vi "fft_demodulator.vi"(0 "Reset":bool, 5 "Config":T2={"IO params"={"Conversion"={"Rate"=4.0, "In channels"=2, "Out channels"=4}, "Carriers"={"Phase shift"=180.0, "Levels"=[[0.8, 0.8, 0.8], [0.03, 0.03, 0.03]], "Delay samples"=73.15}}, "High rate STFT"={"Win param"=101.5, "Window type"=61, "Win order"=2, "DFT size"=64, "Channels"=[7], "Oversample"=64}, "Low rate STFT"={"Win param"=120.0, "Window type"=61, "Win order"=8, "DFT size"=64, "Channels"=[7], "Oversample"=64}, "Filtering"={"Hum"={"Frequency"=0.0, "Tc"=0.0, "Limit"=101.5, "FFT filter"=FALSE, "Detrend mode"=enum."Robust linear", "Enable"=FALSE}, "Kalman"={"Process noise"=101.5, "Measure noise"=101.5, "Unlock m noise"=101.5, "Mode"=enum."FFT"}, "Distortion"={"LF cut"=101.5, "Tc"=3.0, "Limit"=101.5, "FFT filter"=FALSE, "Detrend mode"=enum."Robust linear", "Enable"=FALSE}, "Lowpass"={"Frequency"=0.0, "Order"=0, "Enable"=FALSE}, "Impulse"={"Win order"=102, "Locked limit"=101.5, "Locked count"=102, "Threshold Tc"=101.5, "Thresh sigmas"=101.5, "Thresh min"=101.5, "After"=0, "Detrend"=FALSE, "Enable"=FALSE}}} {"Filtering"."Impulse"."Thresh min" format="%#_3p"; "Filtering"."Impulse"."Threshold Tc" format="%#_3p"; "Filtering"."Impulse"."Locked limit" format="%#_3p"; "Filtering"."Impulse"."Thresh sigmas" format="%#_3p"; "Filtering"."Lowpass"."Frequency" format="%#_4p"; "Filtering"."Distortion"."Limit" format="%#_3p"; "Filtering"."Distortion"."LF cut" format="%#_3p"; "Filtering"."Kalman"."Unlock m noise" format="%#_3p"; "Filtering"."Kalman"."Measure noise" format="%#_3p"; "Filtering"."Kalman"."Process noise" format="%#_3p"; "Filtering"."Hum"."Limit" format="%#_3p"; "Filtering"."Hum"."Frequency" format="%#_4p"; "Low rate STFT"."Oversample" min=1 step=1; "Low rate STFT"."Channels" min=0 step=1; "Low rate STFT"."DFT size" min=1 step=1; "Low rate STFT"."Window type" items=["Rectangle"=0, "Hanning"=1, "Hamming"=2, "Blackman-Harris"=3, "Exact Blackman"=4, "Blackman"=5, "Flat Top"=6, "4 Term B-Harris "=7, "7 Term B-Harris"=8, "Low Sidelobe"=9, "Blackman Nuttall"=11, "Triangle"=30, "Bartlett-Hanning"=31, "Bohman"=32, "Parzen"=33, "Welch"=34, "Kaiser"=60, "Dolph-Chebyshev"=61, "Gaussian"=62]; "High rate STFT"."Oversample" min=1 step=1; "High rate STFT"."Channels" min=0 step=1; "High rate STFT"."DFT size" min=1 step=1; "High rate STFT"."Window type" items=["Rectangle"=0, "Hanning"=1, "Hamming"=2, "Blackman-Harris"=3, "Exact Blackman"=4, "Blackman"=5, "Flat Top"=6, "4 Term B-Harris "=7, "7 Term B-Harris"=8, "Low Sidelobe"=9, "Blackman Nuttall"=11, "Triangle"=30, "Bartlett-Hanning"=31, "Bohman"=32, "Parzen"=33, "Welch"=34, "Kaiser"=60, "Dolph-Chebyshev"=61, "Gaussian"=62]; "IO params"."Carriers"."Levels" min=0.0 step=0.1; "IO params"."Conversion"."Rate" format="%#_8g"}, 7 "Modulation info":T8={"Fs full"=0.0, "Fs high"=0.0, "Fs low"=0.0, "Read size"=0, "FFT size low"=5000, "df low"=5000.0, "High carriers"=[], "Low carriers"=[], "Hi channels at low"=[7]} {"Hi channels at low" min=0 step=1; "Low carriers" format="%#_6p"; "High carriers" format="%#_6p"}, 9 "Low carrier amplitudes":cdb[](array[numeric]) format="%#_3p", 12 "Raw data":dbl[](array[numeric])) -> (10 "High carrier amplitudes":cdb[][](array[numeric]) format="%_3p", 14 "Filtered signal":dbl[](array[numeric]), 15 "Trace channel out":T1)   [LabVIEW 2014]
uses:
  modulation_info.ctl
  ilemt_config.ctl
  IO_params.ctl
  stft_params.ctl
  <vilib>/Analysis/4window.llb/windowTd.ctl
  filter_params.ctl
  detrend_mode.ctl
  trace_channel.ctl
  <vilib>/Analysis/NI_AALPro.lvlib
panel:
  out "DIstortion filter attenuation":dbl
  out "Distortion filter RMS":dbl[](array[numeric])
  out "KF result":cdb[](array[numeric]) format="%_3p"
  out "Distortion filter":dbl[][](graph)
  # "This VI deals with high-rate demodulation and filtering for a single sensor axis."
  # "Rows are time (high carrier samples), columns are high rate source XYZ axis amplitudes."
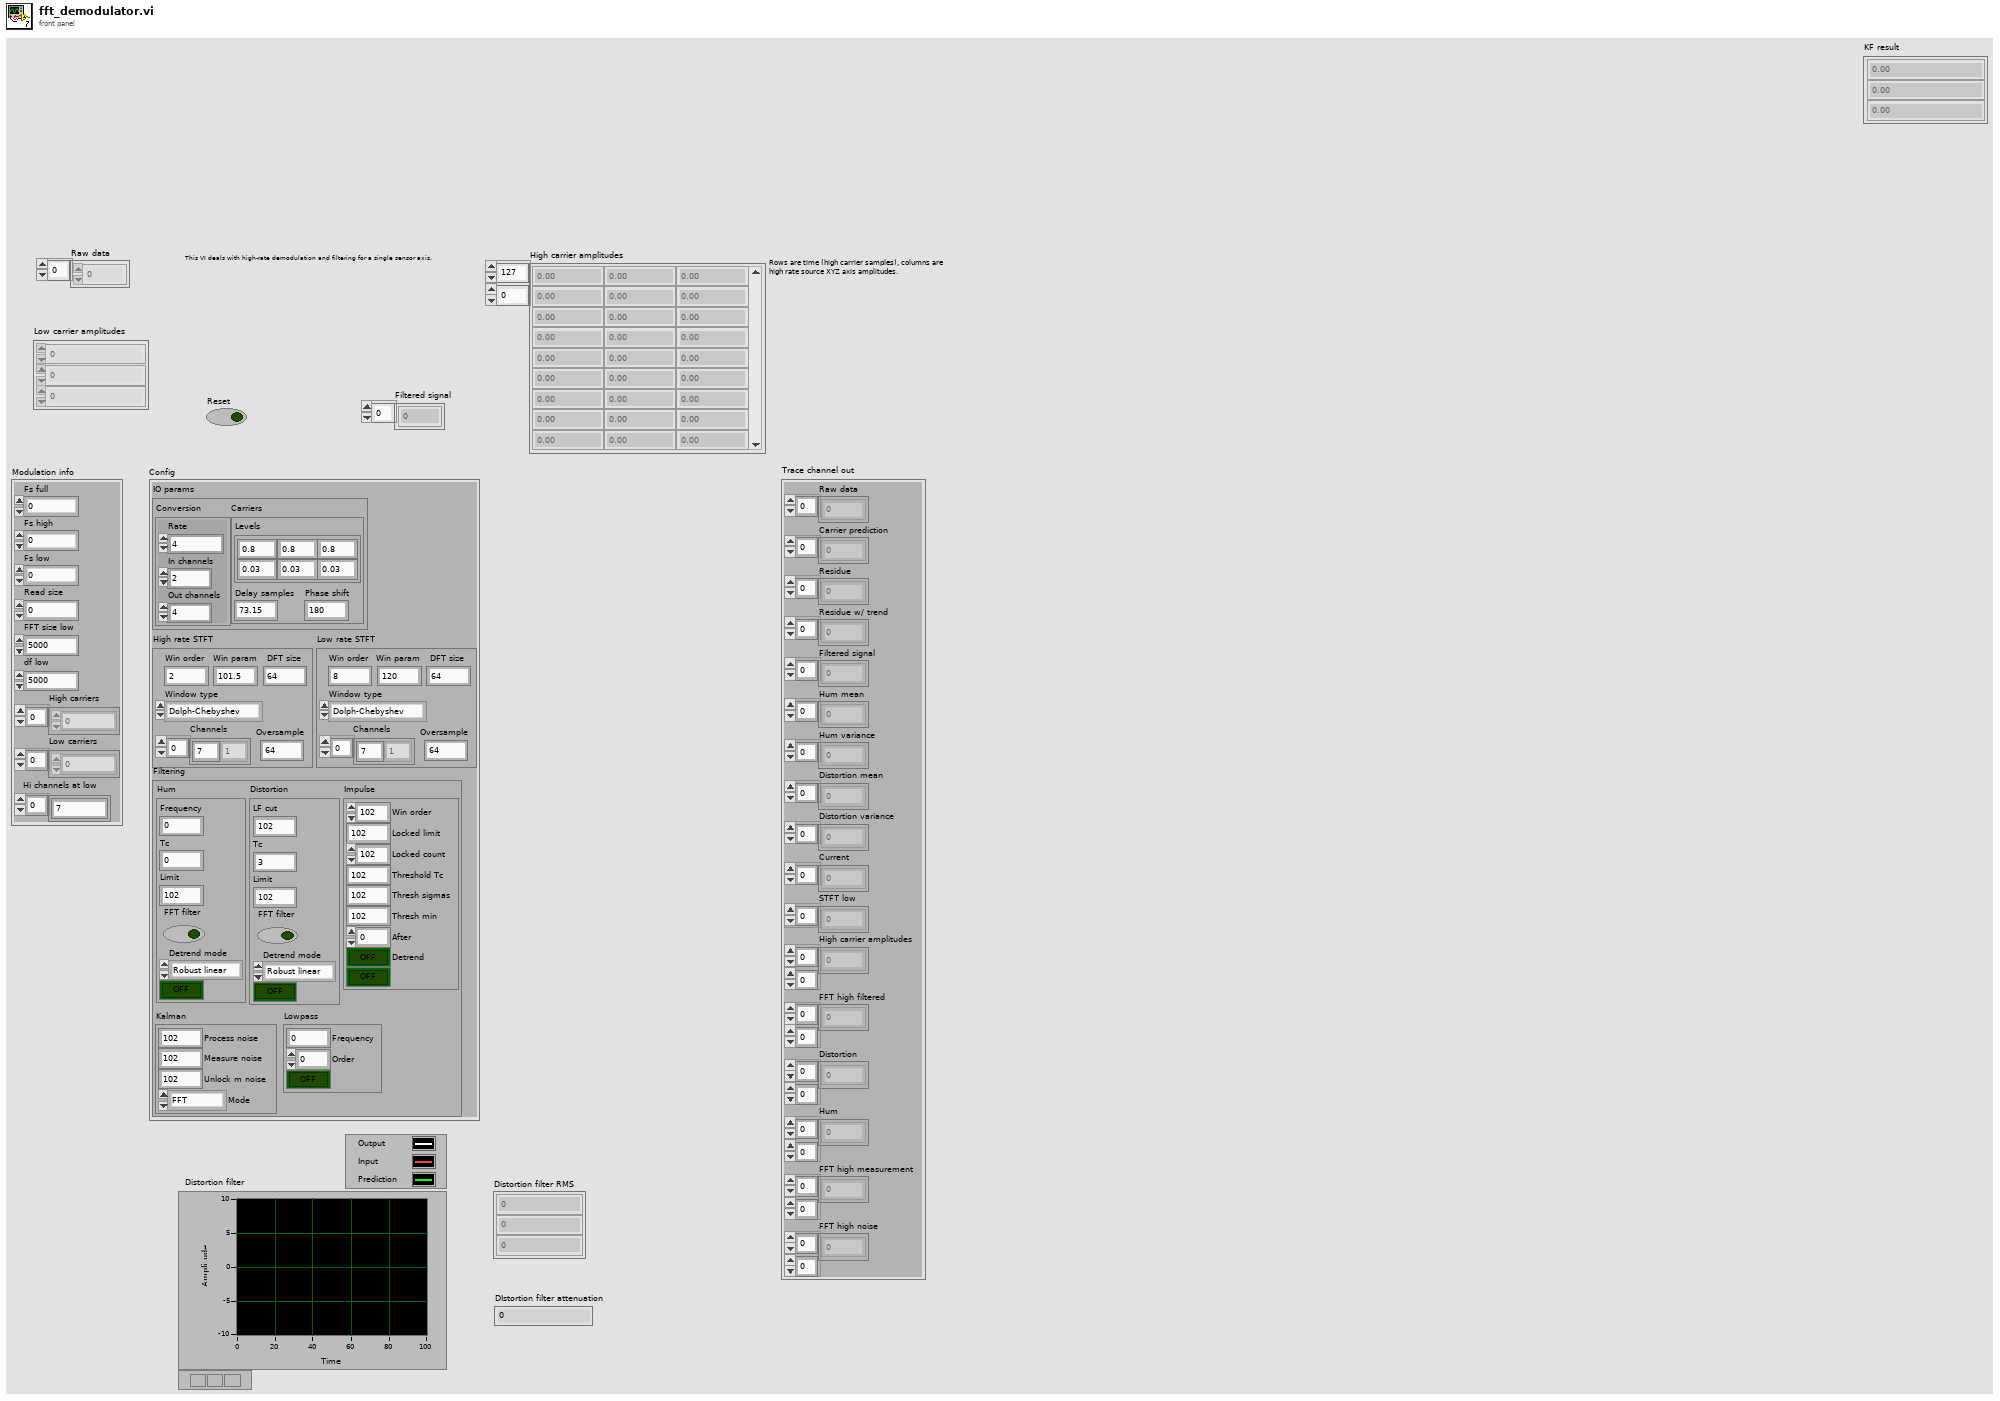
[diagram p1: front panel]
types:
  T1 = typedef "trace_channel.ctl" = cluster{"Raw data":dbl[], "Carrier prediction":dbl[], "Residue":dbl[], "Residue w/ trend":dbl[], "Filtered signal":dbl[], "Hum mean":dbl[], "Hum variance":dbl[], "Distortion mean":dbl[], "Distortion variance":dbl[], "Current":dbl[], "STFT low":cdb[], "High carrier amplitudes":cdb[][], "FFT high filtered":cdb[][], "Distortion":cdb[][], "Hum":cdb[][], "FFT high measurement":cdb[][], "FFT high noise":dbl[][]}
  T2 = typedef "ilemt_config.ctl" = cluster{"IO params":T3, "High rate STFT":T4, "Low rate STFT":T4, "Filtering":T6}
  T3 = typedef "IO_params.ctl" = cluster{"Conversion":cluster{"Rate":dbl, "In channels":u32, "Out channels":u32}, "Carriers":cluster{"Phase shift":dbl, "Levels":dbl[][], "Delay samples":dbl}}
  T4 = typedef "stft_params.ctl" = cluster{"Win param":dbl, "Window type":T5, "Win order":i32, "DFT size":i32, "Channels":i32[], "Oversample":i32}
  T5 = typedef "NI_AALPro.lvlib/windowTd.ctl" = u32
  T6 = typedef "filter_params.ctl" = cluster{"Hum":cluster{"Frequency":dbl, "Tc":dbl, "Limit":dbl, "FFT filter":bool, "Detrend mode":T7, "Enable":bool}, "Kalman":cluster{"Process noise":dbl, "Measure noise":dbl, "Unlock m noise":dbl, "Mode":enum16{"FFT", "KF demod"}}, "Distortion":cluster{"LF cut":dbl, "Tc":dbl, "Limit":dbl, "FFT filter":bool, "Detrend mode":T7, "Enable":bool}, "Lowpass":cluster{"Frequency":dbl, "Order":i32, "Enable":bool}, "Impulse":cluster{"Win order":i32, "Locked limit":dbl, "Locked count":i32, "Threshold Tc":dbl, "Thresh sigmas":dbl, "Thresh min":dbl, "After":i32, "Detrend":bool, "Enable":bool}}
  T7 = typedef "detrend_mode.ctl" = enum16{"Zero mean", "Linear", "Robust linear"}
  T8 = typedef "modulation_info.ctl" = cluster{"Fs full":dbl, "Fs high":dbl, "Fs low":dbl, "Read size":i32, "FFT size low":i32, "df low":dbl, "High carriers":dbl[], "Low carriers":dbl[], "Hi channels at low":i32[]}
  T9 = typedef "averaging_filter_params.ctl" = cluster{"Order":i32, "Time constant":dbl, "Detrend mode":T7, "TD amplitude limit":dbl, "FFT filter":bool, "Notch channels":i32[], "LF cutoff":i32, "FD amplitude limit":dbl}
  T10 = typedef "kalman_filter.ctl" = cluster{"A":T11, "B":T11, "H":T11, "Q":T11, "R":T11, "x":T11, "P":T11, "x lim":dbl[], "y lim":dbl[], "K":T11, "Converge count":i32}
  T11 = typedef "NI_Matrix.lvlib/RealMatrix.ctl" = dbl[][]
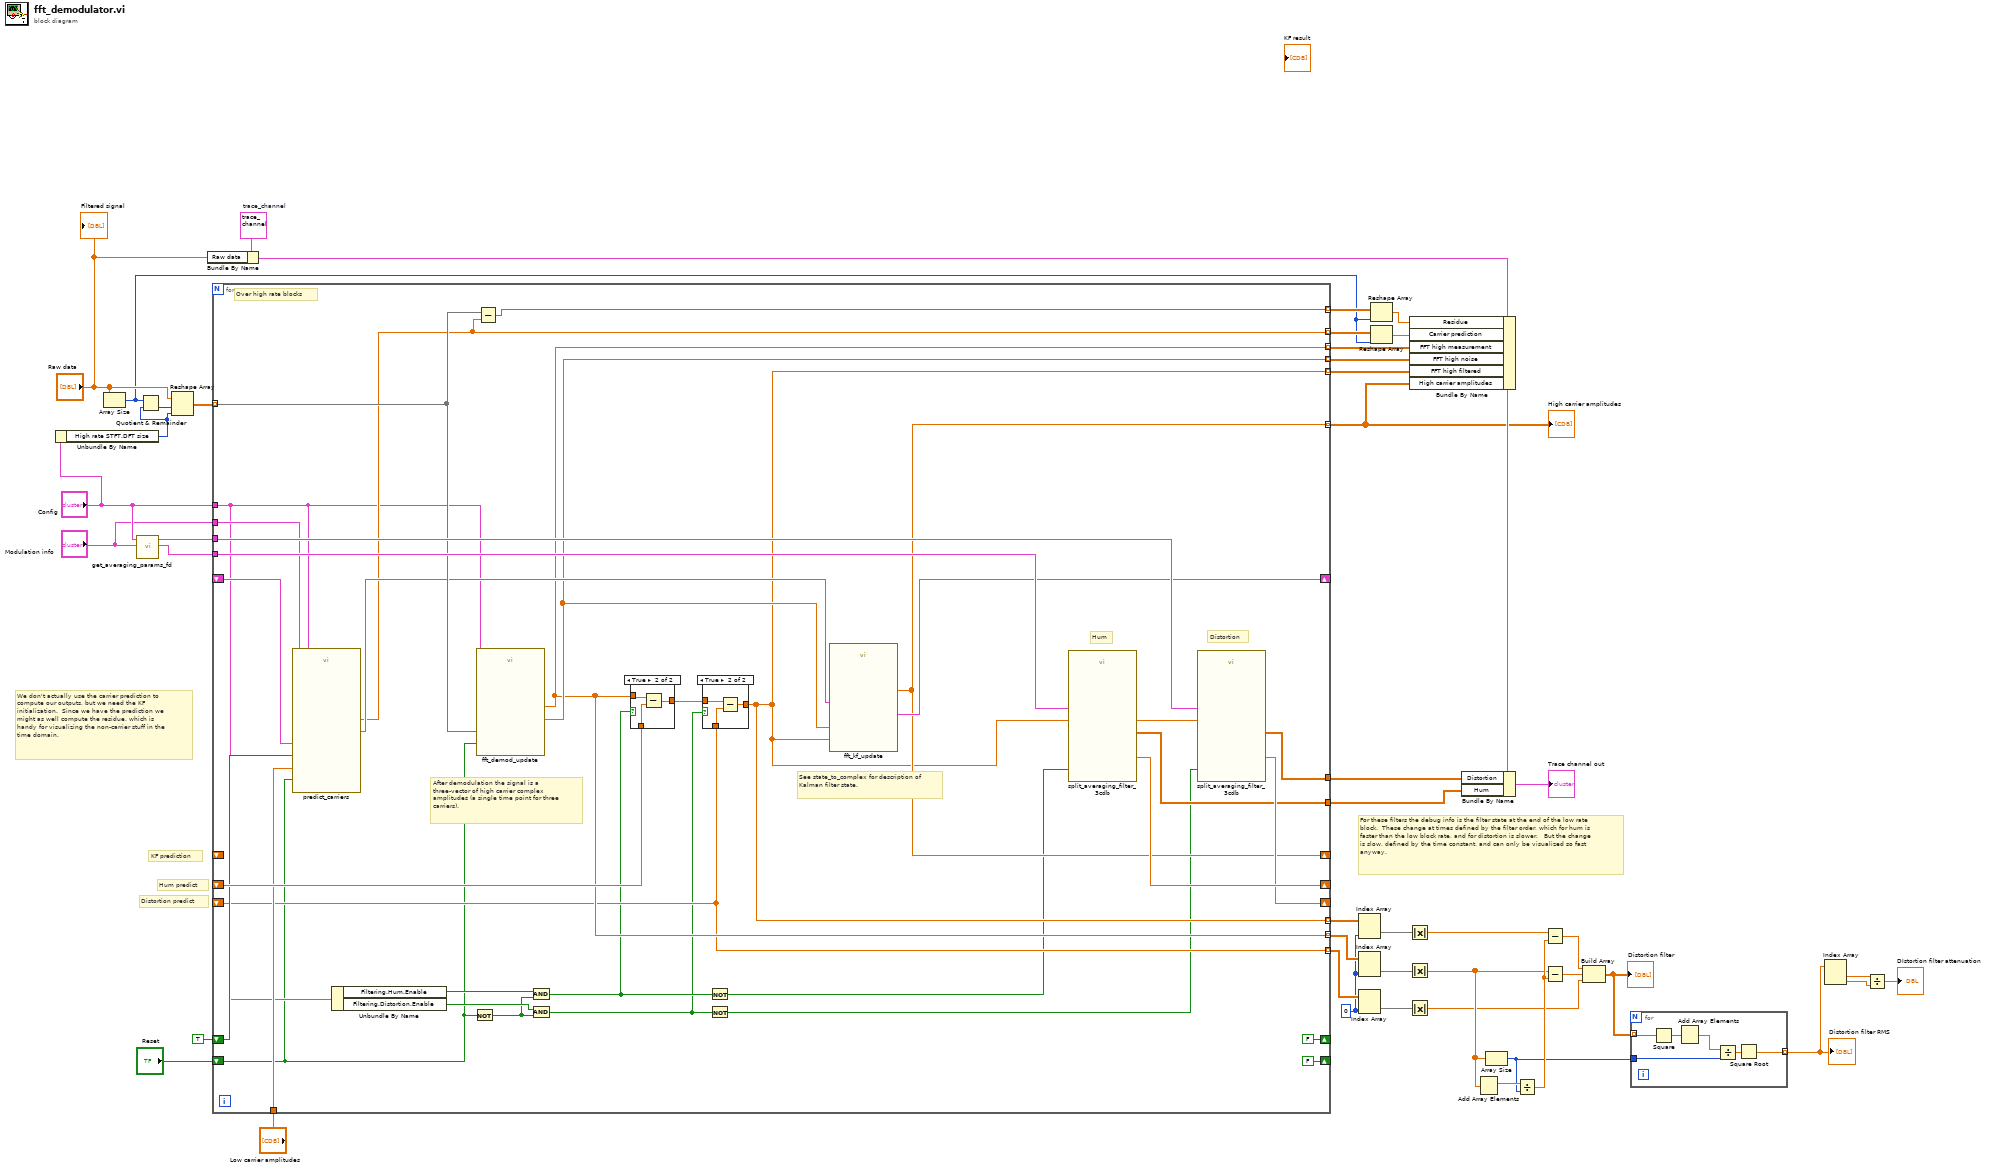
[diagram p0: block diagram]
diagram:
  w15 = 0 ("disabled index (col)")
  w36 = T1 {"Raw data"=[], "Carrier prediction"=[], "Residue"=[], "Residue w/ trend"=[], "Filtered signal"=[], "Hum mean"=[], "Hum variance"=[], "Distortion mean"=[], "Distortion variance"=[], "Current"=[], "STFT low"=[], "High carrier amplitudes"=[], "FFT high filtered"=[], "Distortion"=[], "Hum"=[], "FFT high measurement"=[], "FFT high noise"=[]}  # trace_channel
  # "KF prediction"
  # "We don't actually use the carrier prediction to compute our outputs, but we need the KF initialization.  Since we have the prediction we might as well compute the residue, which is handy for visualizing the non-carrier stuff in the time domain."
  # "For these filters the debug info is the filter state at the end of the low rate block.  These change at times defined by the filter order, which for hum is faster than the low block rate, and for distortion is slower.   But the change is slow, defined by the time constant, and can only be visualized so fast anyway."
  # "Distortion predict"
  # "Hum predict"
  n1 = Unbundle By Name("Config") -> ("High rate STFT.DFT size"=w39:i32)
  n2 = Array Size(array="Raw data") -> (size(s)=w26:i32)
  n3 = call "get_averaging_params_fd.vi"("Modulation info"="Modulation info", "Config"="Config") -> ("Hum params"=w44:T9, "Distortion params"=w46:T9)  [unwired: 8 in]
  n4 = Quotient & Remainder(x=w26, y=w39) -> (floor(x/y)=w42:i32)  [unwired: 1 out]
  n5 = Reshape Array("Raw data", w42, w39) -> (w43:dbl[][])
  n6 = Bundle By Name(cluster=w36, "Raw data"="Raw data") -> (w35:T1)
  n7 = for {
    tunnel: w46 -> [w78]
    tunnel: w43 -> [w66] mode=indexing
    tunnel: w44 -> [w77]
    shift-right: [FALSE ("Reset")] -> _
    shift-left: "Reset" -> [w49]
    shift-right: [w63] -> _
    shift-left: _ -> [w70]
    tunnel: "Config" -> [w55]
    tunnel: [w60] -> w32 mode=indexing
    shift-right: [w76] -> _
    shift-left: _ -> [w74]
    shift-right: [w75] -> _
    shift-left: _ -> [w56]
    tunnel: "Modulation info" -> [w71]
    tunnel: [w73] -> w24
    tunnel: [w72] -> w23
    tunnel: [w59] -> w33 mode=indexing
    shift-right: [FALSE ("Reset")] -> _
    shift-left: TRUE ("Reset") -> [w69]
    tunnel: "Low carrier amplitudes" -> [w67]
    tunnel: [w65] -> w29 mode=indexing
    tunnel: [w61] -> w27 mode=indexing
    tunnel: [w58] -> w22 mode=indexing
    tunnel: [w62] -> w21 mode=indexing
    tunnel: [w56] -> w18 mode=indexing
    tunnel: [w58] -> w17 mode=indexing
    shift-right: [w60] -> _
    shift-left: _ -> [_]
    tunnel: [w59] -> w16 mode=indexing
    # "After demodulation the signal is a three-vector of high carrier complex amplitudes (a single time point for three carriers)."
    # "See state_to_complex for description of Kalman filter state."
    # "Over high rate blocks"
    # "Distortion"
    # "Hum"
    n8 = call "predict_carriers.vi"("Modulation info"=w71, "Low rate block start"=w69, "Low carrier amplitudes"=w67, "KF in"=w70, "Reset"=w49, "Config"=w55) -> ("KF out"=w64:T10, "Predicted carriers"=w61:dbl[])  [unwired: 4 in]
    n9 = Unbundle By Name(w55) -> ("Filtering.Hum.Enable"=w54:bool, "Filtering.Distortion.Enable"=w53:bool)
    n10 = Not(x=w49) -> (.not. x?=w52:bool)
    n11 = call "fft_demod_update.vi"("Reset"=w49, "Config"=w55, "Signal"=w66) -> ("Measure noise covariance"=w62:dbl[], "Measurement amplitudes"=w58:cdb[])  [unwired: 7 in]
    n12 = Subtract(x=w66, y=w61) -> (x-y=w65:dbl[])
    n13 = And(x=w54, y=w52) -> (x .and. y?=w51:bool)
    n14 = And(x=w53, y=w52) -> (x .and. y?=w50:bool)
    n15 = case shown="True" w51 {
      tunnel: [w84 w87] -> w57
      tunnel: w74 -> [_ w86]
      tunnel: w58 -> [w84 w85]
      frame False {
      }
      frame True {
        n16 = Subtract(x=w85, y=w86) -> (x-y=w87:cdb[])
      }
    }
    n17 = case shown="True" w50 {
      tunnel: w57 -> [w80 w83]
      tunnel: w56 -> [_ w82]
      tunnel: [w80 w81] -> w59
      frame False {
      }
      frame True {
        n18 = Subtract(x=w83, y=w82) -> (x-y=w81:cdb[])
      }
    }
    n19 = Not(x=w51) -> (.not. x?=w47:bool)
    n20 = Not(x=w50) -> (.not. x?=w48:bool)
    n21 = call "fft_kf_update.vi"("Measurement"=w59, "Measure noise covariance"=w62, "KF in"=w64) -> ("KF out"=w63:T10, "KF estimate"=w60:cdb[])  [unwired: 7 in]
    n22 = call "split_averaging_filter_3cdb.vi"("Reset"=w47, "Parameters"=w77, "Error"=w59) -> ("Model"=w72:cdb[][], "Prediction"=w76:cdb[])  [unwired: 7 in]
    n23 = call "split_averaging_filter_3cdb.vi"("Reset"=w48, "Parameters"=w78, "Error"=w59) -> ("Model"=w73:cdb[][], "Prediction"=w75:cdb[])  [unwired: 7 in]
  }
  "High carrier amplitudes" <- w32
  n24 = Index Array(array=w16, index (col)=w15) -> (element=w10:cdb[])  [unwired: 1 in]
  n25 = Index Array(array=w17, index (col)=w15) -> (element=w9:cdb[])  [unwired: 1 in]
  n26 = Index Array(array=w18, index (col)=w15) -> (element=w7:cdb[])  [unwired: 1 in]
  n27 = Reshape Array(w29, w26) -> (w28:dbl[])
  n28 = Reshape Array(w27, w26) -> (w25:dbl[])
  n29 = Absolute Value(x=w10) -> (abs(x)=w5:dbl[])
  n30 = Absolute Value(x=w9) -> (abs(x)=w8:dbl[])
  n31 = Absolute Value(x=w7) -> (abs(x)=w6:dbl[])
  n32 = Bundle By Name(cluster=w35, "Residue"=w28, "Carrier prediction"=w25, "FFT high measurement"=w22, "FFT high noise"=w21, "FFT high filtered"=w33, "High carrier amplitudes"=w32) -> (w38:T1)
  n33 = Bundle By Name(cluster=w38, "Distortion"=w24, "Hum"=w23) -> (→"Trace channel out":T1)
  n34 = Add Array Elements(numeric array=w8) -> (sum=w20:dbl)
  n35 = Array Size(array=w8) -> (size(s)=w11:i32)
  n36 = Divide(x=w20, y=w11) -> (x/y=w14:dbl)
  n37 = Subtract(x=w5, y=w14) -> (x-y=w13:dbl[])
  n38 = Subtract(x=w8, y=w14) -> (x-y=w19:dbl[])
  n39 = Build Array(w13, w19, w6) -> (w12:dbl[][])
  "Distortion filter" <- w12
  n40 = for {
    tunnel: w12 -> [w92] mode=indexing
    tunnel: w11 -> [w90]
    tunnel: [w88] -> w4 mode=indexing
    n41 = Square(x=w92) -> (x^2=w91:dbl[])
    n42 = Add Array Elements(numeric array=w91) -> (sum=w93:dbl)
    n43 = Divide(x=w93, y=w90) -> (x/y=w89:dbl)
    n44 = Square Root(x=w89) -> (sqrt(x)=w88:dbl)
  }
  "Distortion filter RMS" <- w4
  n45 = Index Array(array=w4) -> (element #1=w2:dbl, element #2=w1:dbl)  [unwired: 2 in]
  n46 = Divide(x=w2, y=w1) -> (x/y=→"DIstortion filter attenuation":dbl)
  "Filtered signal" <- "Raw data"
